vi "Setup.vi"(10 "Queue Actor":refnum<class "Queue Actor.lvclass">, 11 "Dev Actor in":refnum<class "Dev Actor.lvclass">) -> (3 "Dev Actor out":refnum<class "Dev Actor.lvclass">)   [LabVIEW 2021, in "Dev Actor.lvlib" / "Dev Actor.lvclass"]
uses:
  Dev Actor.lvclass
  Queue Actor/Queue Actor.lvclass
  Dev Actor.lvclass/Dev Actor.ctl
  Dev Panel/Dev Panel.lvclass
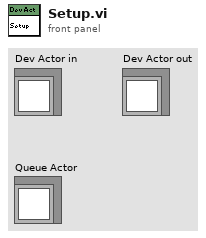
[diagram p1: front panel]
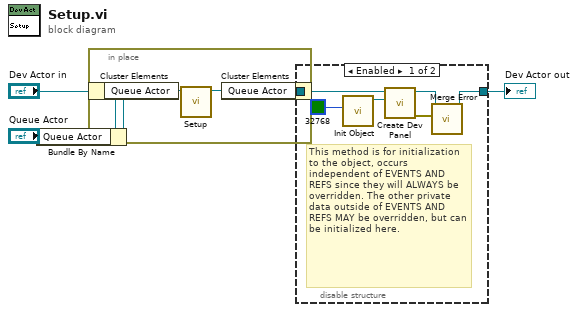
[diagram p0: block diagram]
diagram:
  n1 = Bundle By Name(cluster="Dev Actor in", "Queue Actor"="Queue Actor") -> (w4:refnum<class "Dev Actor.lvclass">)
  n2 = in-place {
    n3 = in-place-cluster #1(w4) -> ("Queue Actor"=w7:refnum<class "Queue Actor.lvclass">)
    n4 = call-dynamic "Setup.vi"("Queue Actor in"=w7) -> ("Queue Actor out"=w6:refnum<class "Queue Actor.lvclass">)  [unwired: 10 in]
    n5 = in-place-cluster #1("Queue Actor"=w6) -> (w2:refnum<class "Dev Actor.lvclass">)
  }
  n6 = disable-structure shown="Enabled" {
    disable-tunnel: w2 -> [w13 _]
    disable-tunnel: [w9 _] -> w1
    frame Enabled {
      # "This method is for initialization to the object, occurs independent of EVENTS AND REFS since they will ALWAYS be overridden. The other private data outside of EVENTS AND REFS MAY be overridden, but can be initialized here."
      n7 = call "Init Object.vi"("BG Color"=u32 32768) -> ("Dev Panel out"=w12:refnum<class "Dev Panel.lvclass">)  [unwired: 10 in]
      n8 = call "Create Dev Panel.vi"("Dev Panel"=w12, "Dev Actor in"=w13) -> ("error out"=w8:errorcluster, "Dev Actor out"=w10:refnum<class "Dev Actor.lvclass">)  [unwired: 8 in]
      n9 = call-dynamic "Merge Error.vi"("Error"=w8, "Dev Actor in"=w10) -> ("Dev Actor out"=w9:refnum<class "Dev Actor.lvclass">)  [unwired: 9 in]
    }
    frame Disabled {
    }
  }
  "Dev Actor out" <- w1
